vi "Fit VI window to Rect.vi"(4 "error in (no error)":errorcluster, 6 "Rect":T1, 7 "VI Ref (calling VI)":refnum<vi>) -> (0 "error out":errorcluster, 3 "VI Ref out":refnum<vi>)   [LabVIEW 2017]
doc: "Resizes and centres the VI window so that it fits inside Rect."
uses:
  <vilib>/Utility/miscctls.llb/LVRectTypeDef.ctl
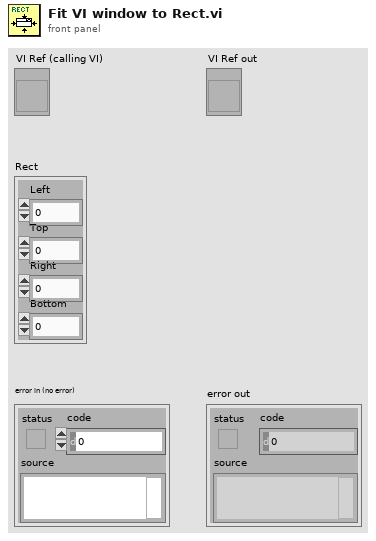
[diagram p1: front panel]
types:
  T1 = typedef "LVRectTypeDef.ctl" = cluster{"Left":i16, "Top":i16, "Right":i16, "Bottom":i16}
  T2 = cluster{"left":i16, "top":i16, "right":i16, "bottom":i16}
  T3 = typedef "LVAllMonitorsDisplayTypeDef.ctl" = cluster{"Bounds":cluster{"Left":i16, "Top":i16, "Right":i16, "Bottom":i16}, "Depth":i16}[]
  T4 = cluster{"Left":i16, "Top":i16, "Right":i16, "Bottom":i16}
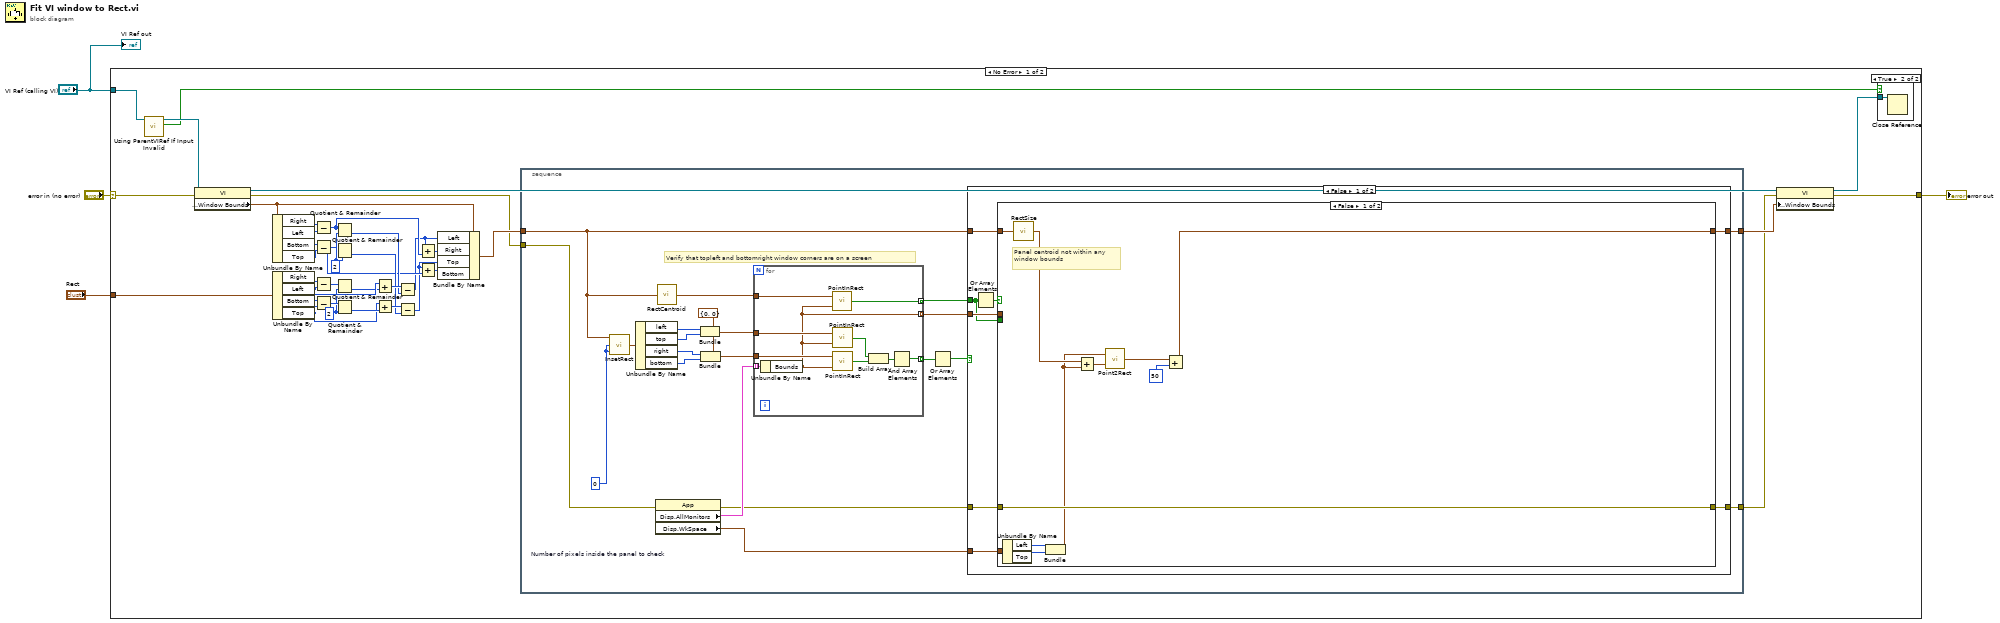
[diagram p0: block diagram]
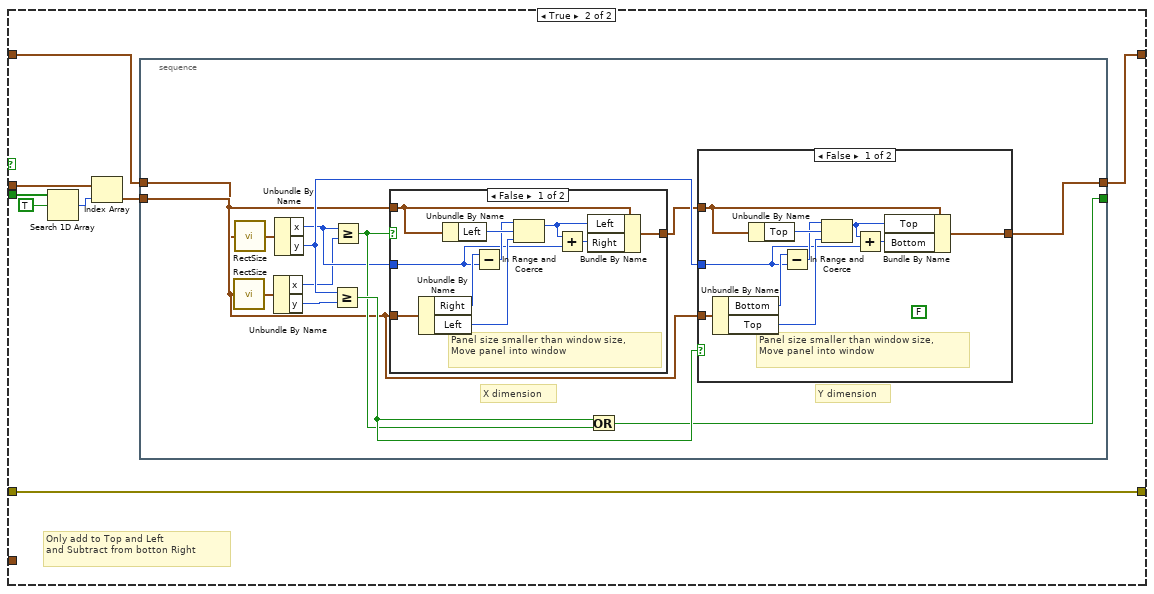
[diagram p2: hidden frame]
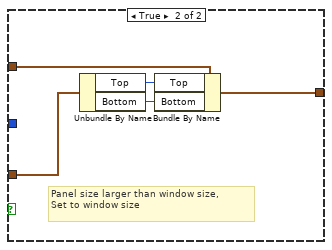
[diagram p3: hidden frame]
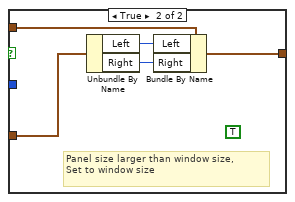
[diagram p4: hidden frame]
diagram:
  n1 = case shown="No Error" "error in (no error)" {
    selector: "error in (no error)" -> [w6 w146]
    tunnel: [w41 w146] -> w4
    tunnel: "VI Ref (calling VI)" -> [w19 _]
    tunnel: "Rect" -> [w5 _]
    frame No Error {
      w36 = i16 2 ("y")
      w20 = i16 2 ("y")
      n2 = call "Using ParentVIRef If Input Invalid.vi"("VI Ref (calling VI)"=w19) -> ("Using Parent Ref(Need to Destroy)"=w9:bool, "VI Ref"=w17:refnum<vi>)  [unwired: 5 in]
      n3 = property class="VI"(reference=w17, error in=w6) -> (reference out=w23:refnum<vi>, error out=w8:errorcluster, "Front Panel Window:Window Bounds"=w12:T1)
      n4 = Unbundle By Name(w12) -> ("Right"=w32:i16, "Left"=w33:i16, "Bottom"=w34:i16, "Top"=w35:i16)
      n5 = Unbundle By Name(w5) -> ("Right"=w40:i16, "Left"=w31:i16, "Bottom"=w39:i16, "Top"=w28:i16)
      n6 = Subtract(x=w32, y=w33) -> (x-y=w22:i16)
      n7 = Subtract(x=w34, y=w35) -> (x-y=w21:i16)
      n8 = Subtract(x=w40, y=w31) -> (x-y=w38:i16)
      n9 = Subtract(x=w39, y=w28) -> (x-y=w37:i16)
      n10 = Quotient & Remainder(x=w22, y=w36) -> (floor(x/y)=w26:i16)  [unwired: 1 out]
      n11 = Quotient & Remainder(x=w21, y=w36) -> (floor(x/y)=w24:i16)  [unwired: 1 out]
      n12 = Quotient & Remainder(x=w38, y=w20) -> (floor(x/y)=w30:i16)  [unwired: 1 out]
      n13 = Quotient & Remainder(x=w37, y=w20) -> (floor(x/y)=w29:i16)  [unwired: 1 out]
      n14 = Add(x=w31, y=w30) -> (x+y=w27:i16)
      n15 = Add(x=w28, y=w29) -> (x+y=w25:i16)
      n16 = Subtract(x=w27, y=w26) -> (x-y=w15:i16)
      n17 = Subtract(x=w25, y=w24) -> (x-y=w14:i16)
      n18 = Add(x=w15, y=w22) -> (x+y=w13:i16)
      n19 = Add(x=w14, y=w21) -> (x+y=w16:i16)
      n20 = Bundle By Name(cluster=w12, "Left"=w15, "Right"=w13, "Top"=w14, "Bottom"=w16) -> (w11:T1)
      n21 = stacked-sequence {
        tunnel: [w52] -> w7
        tunnel: [w43] -> w10
        tunnel: w8 -> [w45]
        tunnel: w11 -> [w59]
        frame #0 {
          w54 = i16 0  # Number of pixels inside the panel to check
          w58 = cluster{"x":i16, "y":i16} {"x"=0, "y"=0} ("point")
          # "Verify that topleft and bottomright window corners are on a screen"
          n22 = call <vilib>:"InsetRect.vi"("dv"=w54, "dh"=w54, "rect"=w59) -> ("inset rect"=w48:T2)
          n23 = Unbundle By Name(w48) -> ("left"=w46:i16, "top"=w47:i16, "right"=w55:i16, "bottom"=w56:i16)
          n24 = property class="App"(error in=w45) -> (error out=w42:errorcluster, "Disp.AllMonitors"=w44:T3, "Disp.WkSpace"=w53:T1)  [unwired: 1 in, 1 out]
          n25 = call <vilib>:"RectCentroid.vi"("rect"=w59) -> ("point"=w60:cluster{"x":i16, "y":i16})
          n26 = Bundle(cluster=w58, "x"=w46, "y"=w47) -> (w49:cluster{"x":i16, "y":i16})
          n27 = Bundle(cluster=w58, "x"=w55, "y"=w56) -> (w57:cluster{"x":i16, "y":i16})
          n28 = for {
            tunnel: w44 -> [w144] mode=indexing
            tunnel: w49 -> [w143]
            tunnel: [w139] -> w50 mode=indexing
            tunnel: w57 -> [w138]
            tunnel: w60 -> [w137]
            tunnel: [w136] -> w61 mode=indexing
            tunnel: [w135] -> w62 mode=indexing
            n29 = Unbundle By Name(w144) -> ("Bounds"=w135:T4)
            n30 = call <vilib>:"PointInRect.vi"("rect"=w135, "point"=w137) -> ("pt in rect"=w136:bool)
            n31 = call <vilib>:"PointInRect.vi"("rect"=w135, "point"=w143) -> ("pt in rect"=w142:bool)
            n32 = call <vilib>:"PointInRect.vi"("rect"=w135, "point"=w138) -> ("pt in rect"=w141:bool)
            n33 = Build Array(w142, w141) -> (w140:bool[])
            n34 = And Array Elements(Boolean array=w140) -> (logical AND=w139:bool)
          }
          n35 = Or Array Elements(Boolean array=w50) -> (logical OR=w51:bool)
          n36 = case shown="False" w51 {
            tunnel: w42 -> [w65 w134]
            tunnel: [w64 w134] -> w52
            tunnel: w59 -> [w69 w133]
            tunnel: [w68 w133] -> w43
            tunnel: w53 -> [w70 _]
            tunnel: w61 -> [w63 _]
            tunnel: w62 -> [w66 _]
            frame False {
              n37 = Or Array Elements(Boolean array=w63) -> (logical OR=w67:bool)
              n38 = case shown="False" w67 {
                tunnel: w70 -> [w81 _]
                tunnel: w69 -> [w77 w84]
                tunnel: [w75 w82] -> w68
                tunnel: w66 -> [_ w86]
                tunnel: w65 -> [w74 w89]
                tunnel: [w74 w89] -> w64
                tunnel: w63 -> [_ w88]
                frame False {
                  # "Panel centroid not within any\nwindow bounds"
                  n39 = Unbundle By Name(w81) -> ("Left"=w80:i16, "Top"=w79:i16)
                  n40 = call <vilib>:"RectSize.vi"("rect"=w77) -> ("point"=w73:cluster{"x":i16, "y":i16})
                  n41 = Bundle("Left"=w80, "Top"=w79) -> (w71:cluster{"Left":i16, "Top":i16})  [unwired: 1 in]
                  n42 = Add(x=w73, y=w71) -> (x+y=w72:cluster{i16, i16})
                  n43 = call <vilib>:"Point2Rect.vi"("point b"=w72, "point a"=w71) -> ("rect"=w76:T2)
                  n44 = Add(x=w76, y=i16 50) -> (x+y=w75:T2)
                }
                frame True {
                  # "Only add to Top and Left\nand Subtract from botton Right"
                  n45 = Search 1D Array(1D array=w88, element=TRUE) -> (index of element=w85:i32)  [unwired: 1 in]
                  n46 = Index Array(array=w86, index=w85) -> (element=w83:T4)
                  n47 = stacked-sequence {
                    tunnel: [w90] -> _
                    tunnel: [w100] -> w82
                    tunnel: w83 -> [w99]
                    tunnel: w84 -> [w91]
                    frame #0 {
                      # "X dimension"
                      # "Y dimension"
                      n48 = call <vilib>:"RectSize.vi"("rect"=w99) -> ("point"=w93:cluster{"x":i16, "y":i16})
                      n49 = call <vilib>:"RectSize.vi"("rect"=w91) -> ("point"=w92:cluster{"x":i16, "y":i16})
                      n50 = Unbundle By Name(w93) -> ("x"=w94:i16, "y"=w97:i16)
                      n51 = Unbundle By Name(w92) -> ("x"=w95:i16, "y"=w98:i16)
                      n52 = Greater Or Equal?(x=w98, y=w97) -> (x >= y?=w102:bool)
                      n53 = Greater Or Equal?(x=w95, y=w94) -> (x >= y?=w101:bool)
                      n54 = case shown="False" w101 {
                        tunnel: w99 -> [w127 w128]
                        tunnel: w91 -> [w119 w129]
                        tunnel: w95 -> [w120 _]
                        tunnel: [w118 w130] -> w96
                        frame False {
                          # "Panel size smaller than window size,\nMove panel into window"
                          n55 = Unbundle By Name(w127) -> ("Right"=w123:i16, "Left"=w125:i16)
                          n56 = Unbundle By Name(w119) -> ("Left"=w126:i16)
                          n57 = Subtract(x=w123, y=w120) -> (x-y=w124:i16)
                          n58 = In Range and Coerce(upper limit=w124, x=w126, lower limit=w125) -> (coerced(x)=w122:i16)  [unwired: 1 out]
                          n59 = Add(x=w122, y=w120) -> (x+y=w121:i16)
                          n60 = Bundle By Name(cluster=w119, "Left"=w122, "Right"=w121) -> (w118:T1)
                        }
                        frame True {
                          (unwired) TRUE
                          # "Panel size larger than window size,\nSet to window size"
                          n61 = Unbundle By Name(w128) -> ("Left"=w132:i16, "Right"=w131:i16)
                          n62 = Bundle By Name(cluster=w129, "Left"=w132, "Right"=w131) -> (w130:T1)
                        }
                      }
                      n63 = Or(x=w102, y=w101) -> (x .or. y?=w90:bool)
                      n64 = case shown="False" w102 {
                        tunnel: w99 -> [w112 w117]
                        tunnel: w96 -> [w104 w113]
                        tunnel: w98 -> [w105 _]
                        tunnel: [w103 w114] -> w100
                        frame False {
                          (unwired) FALSE
                          # "Panel size smaller than window size,\nMove panel into window"
                          n65 = Unbundle By Name(w112) -> ("Bottom"=w108:i16, "Top"=w110:i16)
                          n66 = Unbundle By Name(w104) -> ("Top"=w111:i16)
                          n67 = Subtract(x=w108, y=w105) -> (x-y=w109:i16)
                          n68 = In Range and Coerce(upper limit=w109, x=w111, lower limit=w110) -> (coerced(x)=w107:i16)  [unwired: 1 out]
                          n69 = Add(x=w107, y=w105) -> (x+y=w106:i16)
                          n70 = Bundle By Name(cluster=w104, "Top"=w107, "Bottom"=w106) -> (w103:T1)
                        }
                        frame True {
                          # "Panel size larger than window size,\nSet to window size"
                          n71 = Unbundle By Name(w117) -> ("Top"=w116:i16, "Bottom"=w115:i16)
                          n72 = Bundle By Name(cluster=w113, "Top"=w116, "Bottom"=w115) -> (w114:T1)
                        }
                      }
                    }
                  }
                }
              }
            }
            frame True {
            }
          }
        }
      }
      n73 = property class="VI"(reference=w23, error in=w7, "Front Panel Window:Window Bounds"=w10) -> (reference out=w18:refnum<vi>, error out=w41:errorcluster)
      n74 = case shown="True" w9 {
        tunnel: w18 -> [_ w145]
        frame False {
        }
        frame True {
          n75 = Close Reference(reference=w145) -> ()  [unwired: 1 in, 1 out]
        }
      }
    }
    frame Error {
    }
  }
  "error out" <- w4
  "VI Ref out" <- "VI Ref (calling VI)"
